vi "自动售货机.vi"() -> ()   [LabVIEW 2018]
panel:
  in  "数值 2":dbl
  in  "数值":dbl
  in  "选项卡控件":enum32{"前面板", "后台"}(tab)
  in  "果粒橙":bool
  in  "营养快线":bool
  in  "矿泉水":bool
  in  "花生奶":bool
  in  "绿茶":bool
  in  "雪梨":bool
  in  "红牛":bool
  in  "八宝粥":bool
  in  "王老吉":bool
  in  "可乐":bool
  in  "雪碧":bool
  in  "百事":bool
  in  "退币":bool
  in  "5角":bool
  in  "1元":bool
  in  "5元":bool
  in  "10元":bool
  in  "投币显示":string
  in  "字符串":string
  out "果粒橙":dbl
  out "营养快线":dbl
  out "矿泉水":dbl
  out "花生奶":dbl
  out "绿茶":dbl
  out "雪梨":dbl
  out "红牛":dbl
  out "八宝粥":dbl
  out "王老吉":dbl
  out "可乐":dbl
  out "雪碧":dbl
  out "百事":dbl
  in  "销售金额":string
  in  "关闭售货机":bool
  in  "销售记录":string
  in  "果粒橙单价":dbl
  in  "营养快线数量":dbl
  in  "矿泉水数量":dbl
  in  "花生奶数量":dbl
  in  "绿茶数量":dbl
  in  "雪梨数量":dbl
  in  "红牛数量":dbl
  in  "八宝粥数量":dbl
  in  "王老吉数量":dbl
  in  "可乐数量":dbl
  in  "雪碧数量":dbl
  in  "百事数量":dbl
  in  "果粒橙数量":dbl
  in  "营养快线单价":dbl
  in  "矿泉水单价":dbl
  in  "花生奶单价":dbl
  in  "绿茶单价":dbl
  in  "雪梨单价":dbl
  in  "红牛单价":dbl
  in  "八宝粥单价":dbl
  in  "王老吉单价":dbl
  in  "可乐单价":dbl
  in  "雪碧单价":dbl
  in  "上货":bool
  in  "百事单价":dbl
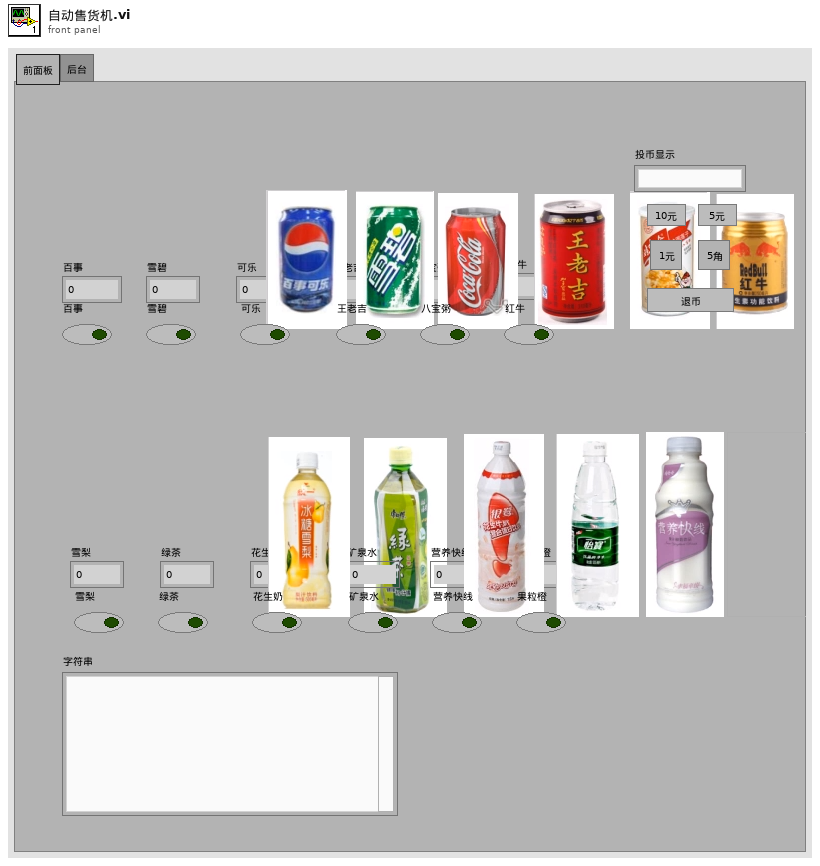
[diagram p1: front panel]
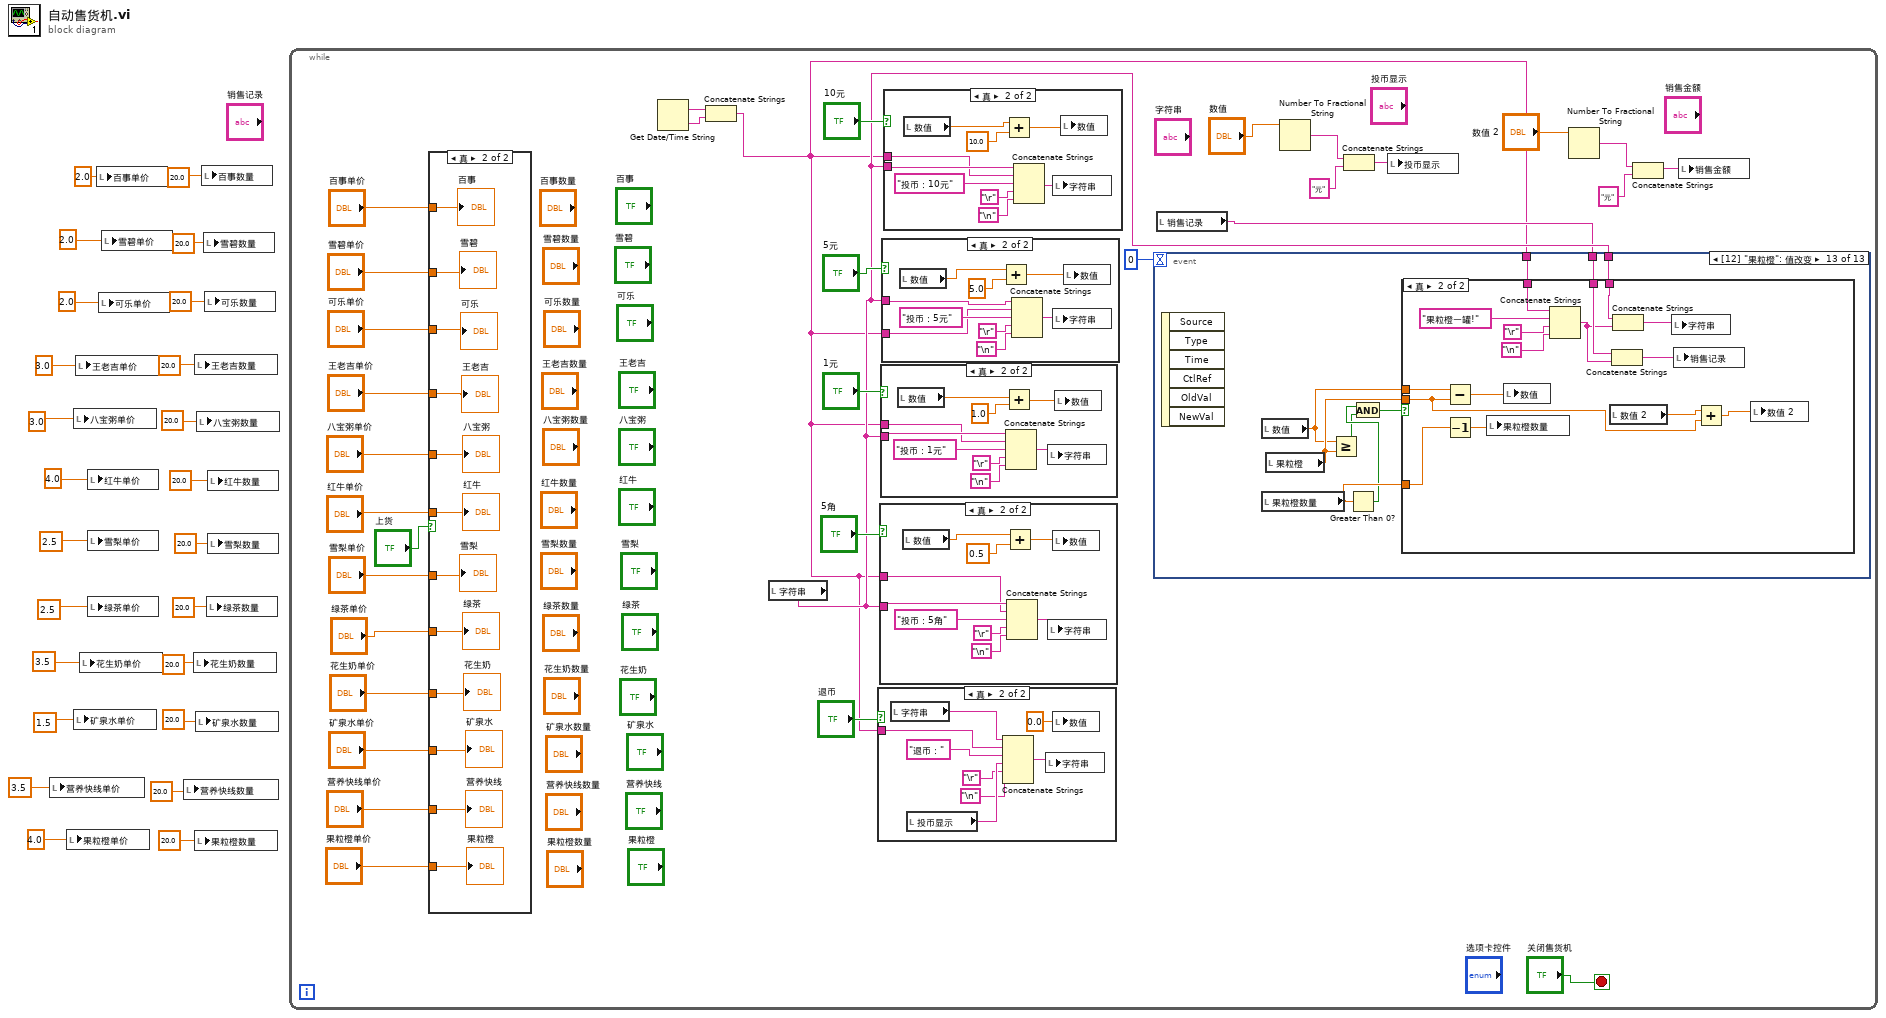
[diagram p0: block diagram]
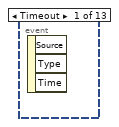
[diagram p2: hidden frame]
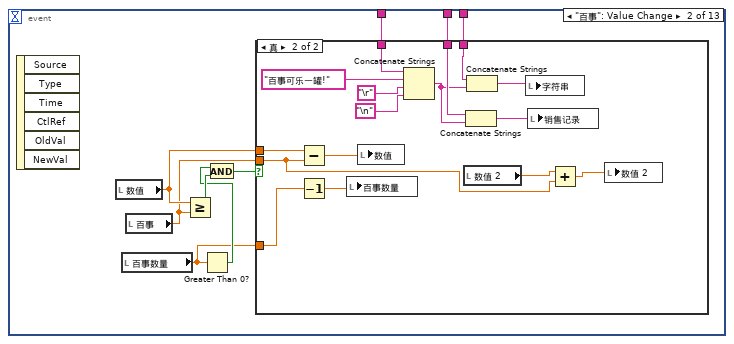
[diagram p3: hidden frame]
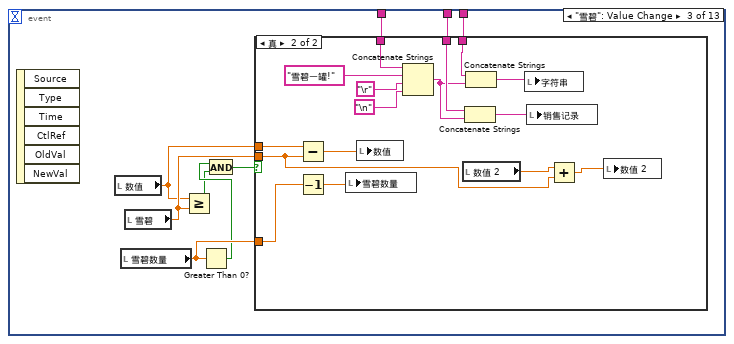
[diagram p5: hidden frame]
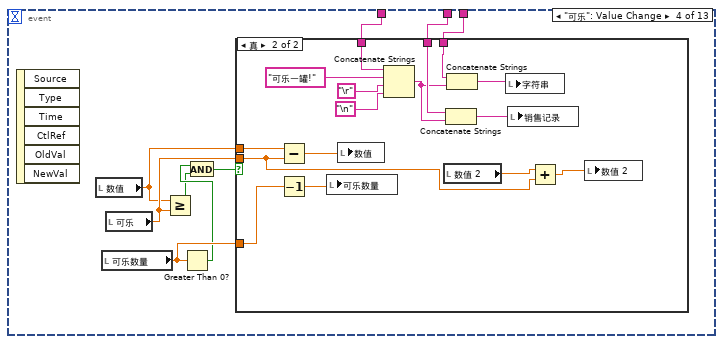
[diagram p7: hidden frame]
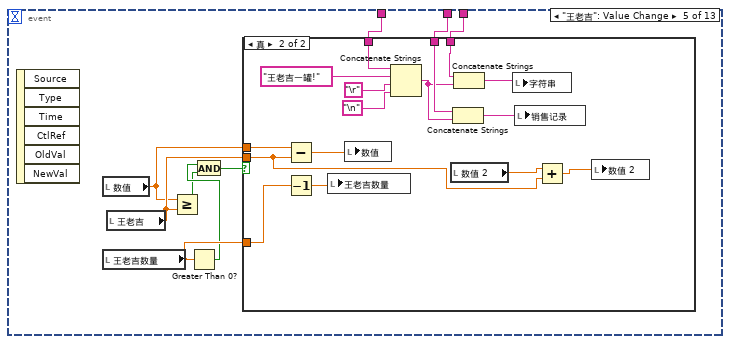
[diagram p9: hidden frame]
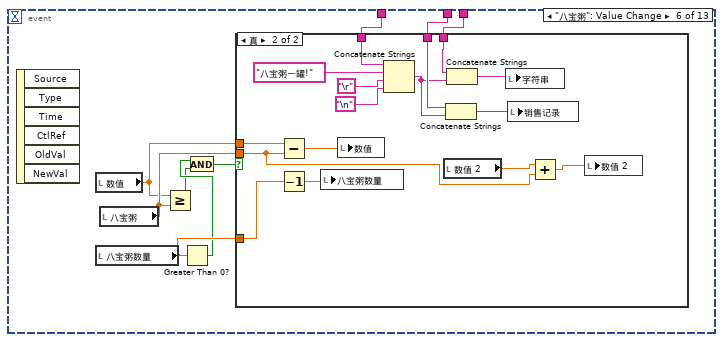
[diagram p11: hidden frame]
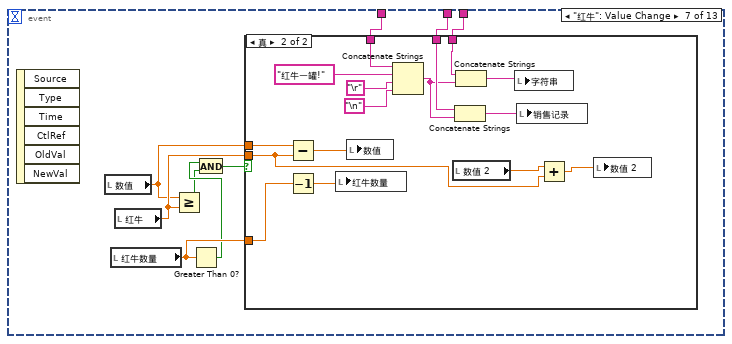
[diagram p13: hidden frame]
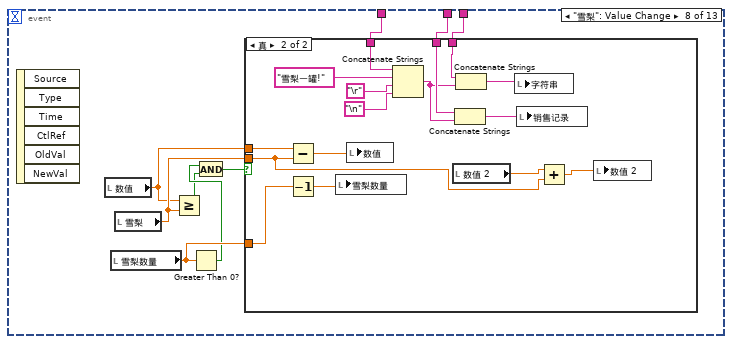
[diagram p15: hidden frame]
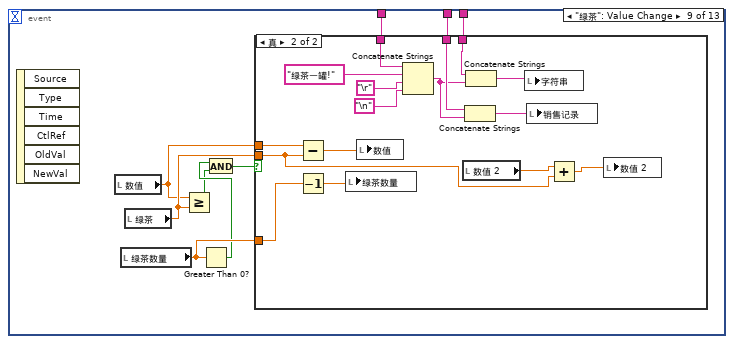
[diagram p17: hidden frame]
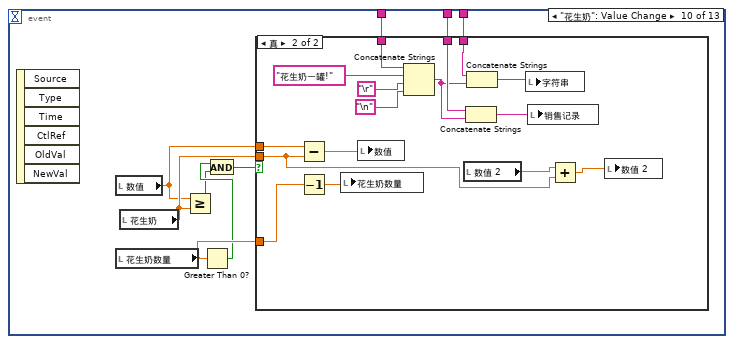
[diagram p19: hidden frame]
diagram:
  n1 = local write "营养快线单价"(3.5 ("百事单价")) -> ()
  n2 = local write "果粒橙单价"(4.0 ("百事单价")) -> ()
  n3 = local write "八宝粥单价"(3.0 ("百事单价")) -> ()
  n4 = local write "矿泉水单价"(1.5 ("百事单价")) -> ()
  n5 = local write "王老吉单价"(3.0 ("百事单价")) -> ()
  n6 = local write "花生奶单价"(3.5 ("百事单价")) -> ()
  n7 = local write "红牛单价"(4.0 ("百事单价")) -> ()
  n8 = local write "雪梨单价"(2.5 ("百事单价")) -> ()
  n9 = local write "绿茶单价"(2.5 ("百事单价")) -> ()
  n10 = local write "百事单价"(2.0 ("百事单价")) -> ()
  n11 = local write "可乐单价"(2.0 ("百事单价")) -> ()
  n12 = local write "雪碧单价"(2.0 ("百事单价")) -> ()
  n13 = local write "营养快线数量"(20.0 ("百事单价")) -> ()
  n14 = local write "花生奶数量"(20.0 ("百事单价")) -> ()
  n15 = local write "王老吉数量"(20.0 ("百事单价")) -> ()
  n16 = local write "果粒橙数量"(20.0 ("百事单价")) -> ()
  n17 = local write "矿泉水数量"(20.0 ("百事单价")) -> ()
  n18 = local write "八宝粥数量"(20.0 ("百事单价")) -> ()
  n19 = local write "百事数量"(20.0 ("百事单价")) -> ()
  n20 = local write "雪碧数量"(20.0 ("百事单价")) -> ()
  n21 = local write "可乐数量"(20.0 ("百事单价")) -> ()
  n22 = local write "绿茶数量"(20.0 ("百事单价")) -> ()
  n23 = local write "红牛数量"(20.0 ("百事单价")) -> ()
  n24 = local write "雪梨数量"(20.0 ("百事单价")) -> ()
  n25 = while {
    stop <- "关闭售货机" stop-if-true
    n26 = case shown="真" "上货" {
      tunnel: "百事单价" -> [_ w413]
      tunnel: "雪碧单价" -> [_ w412]
      tunnel: "可乐单价" -> [_ w411]
      tunnel: "王老吉单价" -> [_ w410]
      tunnel: "八宝粥单价" -> [_ w409]
      tunnel: "红牛单价" -> [_ w408]
      tunnel: "雪梨单价" -> [_ w407]
      tunnel: "绿茶单价" -> [_ w406]
      tunnel: "花生奶单价" -> [_ w405]
      tunnel: "矿泉水单价" -> [_ w404]
      tunnel: "营养快线单价" -> [_ w403]
      tunnel: "果粒橙单价" -> [_ w402]
      frame False {
      }
      frame True {
        "百事" <- w413
        "雪碧" <- w412
        "可乐" <- w411
        "王老吉" <- w410
        "八宝粥" <- w409
        "红牛" <- w408
        "雪梨" <- w407
        "绿茶" <- w406
        "花生奶" <- w405
        "矿泉水" <- w404
        "营养快线" <- w403
        "果粒橙" <- w402
      }
    }
    n27 = Get Date/Time String() -> (date string=w29:string, time string=w28:string)  [unwired: 3 in]
    n28 = Concatenate Strings(w29, w28) -> (w27:string)
    n29 = local read "字符串"() -> (w34:string)
    n30 = case shown="真" "退币" {
      tunnel: w27 -> [_ w358]
      frame False {
      }
      frame True {
        n31 = local read "字符串"() -> (w359:string)
        n32 = local read "投币显示"() -> (w362:string)
        n33 = Concatenate Strings(w359, w358, "退币：" ("字符串"), w362, "\r", "\n") -> (w364:string)
        n34 = local write "字符串"(w364) -> ()
        n35 = local write "数值"(0.0 ("数值")) -> ()
      }
    }
    n36 = case shown="真" "5角" {
      tunnel: w34 -> [_ w367]
      tunnel: w27 -> [_ w366]
      frame False {
      }
      frame True {
        n37 = local read "数值"() -> (w372:dbl)
        n38 = Add(x=w372, y=0.5) -> (x+y=w373:dbl)
        n39 = Concatenate Strings(w367, w366, "投币：5角" ("字符串"), "\r", "\n") -> (w371:string)
        n40 = local write "字符串"(w371) -> ()
        n41 = local write "数值"(w373) -> ()
      }
    }
    n42 = case shown="真" "1元" {
      tunnel: w34 -> [_ w376]
      tunnel: w27 -> [_ w375]
      frame False {
      }
      frame True {
        n43 = local read "数值"() -> (w381:dbl)
        n44 = Add(x=w381, y=1.0) -> (x+y=w382:dbl)
        n45 = Concatenate Strings(w376, w375, "投币：1元" ("字符串"), "\r", "\n") -> (w377:string)
        n46 = local write "字符串"(w377) -> ()
        n47 = local write "数值"(w382) -> ()
      }
    }
    n48 = case shown="真" "5元" {
      tunnel: w34 -> [_ w385]
      tunnel: w27 -> [_ w384]
      frame False {
      }
      frame True {
        n49 = local read "数值"() -> (w390:dbl)
        n50 = Add(x=w390, y=5.0) -> (x+y=w391:dbl)
        n51 = Concatenate Strings(w385, w384, "投币：5元" ("字符串"), "\r", "\n") -> (w386:string)
        n52 = local write "字符串"(w386) -> ()
        n53 = local write "数值"(w391) -> ()
      }
    }
    n54 = case shown="真" "10元" {
      tunnel: w34 -> [_ w394]
      tunnel: w27 -> [_ w393]
      frame False {
      }
      frame True {
        n55 = local read "数值"() -> (w400:dbl)
        n56 = Add(x=w400, y=10.0) -> (x+y=w401:dbl)
        n57 = Concatenate Strings(w394, w393, "投币：10元" ("字符串"), "\r", "\n") -> (w395:string)
        n58 = local write "字符串"(w395) -> ()
        n59 = local write "数值"(w401) -> ()
      }
    }
    n60 = local read "销售记录"() -> (w33:string)
    n61 = event shown="[12] \"果粒橙\": 值改变" {
      selector: _ -> [_ _ _ _ _ _ _ _ _ _ _ _ _]
      dyn-events: _ -> [_ _ _ _ _ _ _ _ _ _ _ _ _]
      timeout: 0 -> [_ _ _ _ _ _ _ _ _ _ _ _ _]
      tunnel: w34 -> [_ w66 w85 w110 w134 w160 w183 w209 w235 w258 w285 w310 w335]
      tunnel: w33 -> [_ w65 w84 w109 w135 w159 w184 w210 w234 w259 w284 w309 w334]
      tunnel: w27 -> [_ w58 w83 w108 w133 w158 w185 w208 w233 w260 w283 w308 w333]
      event Timeout {
        n62 = event-data() -> ()  [unwired: 1 in, 3 out]
      }
      event "百事": Value Change {
        n63 = event-data() -> ()  [unwired: 1 in, 6 out]
        n64 = local read "数值"() -> (w64:dbl)
        n65 = local read "百事数量"() -> (w59:dbl)
        n66 = local read "百事"() -> (w63:dbl)
        n67 = Greater Or Equal?(x=w64, y=w63) -> (x >= y?=w62:bool)
        n68 = Greater Than 0?(x=w59) -> (x > 0?=w60:bool)
        n69 = And(x=w60, y=w62) -> (x .and. y?=w61:bool)
        n70 = case shown="真" w61 {
          tunnel: w66 -> [_ w78]
          tunnel: w65 -> [_ w77]
          tunnel: w64 -> [_ w74]
          tunnel: w63 -> [_ w69]
          tunnel: w59 -> [_ w72]
          tunnel: w58 -> [_ w68]
          frame False {
          }
          frame True {
            n71 = Subtract(x=w74, y=w69) -> (x-y=w75:dbl)
            n72 = Decrement(x=w72) -> (x-1=w73:dbl)
            n73 = local write "百事数量"(w73) -> ()
            n74 = local write "数值"(w75) -> ()
            n75 = Concatenate Strings(w68, "百事可乐一罐!" ("字符串"), "\r", "\n") -> (w76:string)
            n76 = local read "数值 2"() -> (w71:dbl)
            n77 = Concatenate Strings(w77, w76) -> (w67:string)
            n78 = Concatenate Strings(w78, w76) -> (w79:string)
            n79 = local write "字符串"(w79) -> ()
            n80 = local write "销售记录"(w67) -> ()
            n81 = Add(x=w71, y=w69) -> (x+y=w70:dbl)
            n82 = local write "数值 2"(w70) -> ()
          }
        }
      }
      event "雪碧": Value Change {
        n83 = event-data() -> ()  [unwired: 1 in, 6 out]
        n84 = local read "数值"() -> (w86:dbl)
        n85 = local read "雪碧数量"() -> (w91:dbl)
        n86 = local read "雪碧"() -> (w87:dbl)
        n87 = Greater Or Equal?(x=w86, y=w87) -> (x >= y?=w88:bool)
        n88 = Greater Than 0?(x=w91) -> (x > 0?=w90:bool)
        n89 = And(x=w90, y=w88) -> (x .and. y?=w89:bool)
        n90 = case shown="真" w89 {
          tunnel: w85 -> [_ w103]
          tunnel: w84 -> [_ w102]
          tunnel: w86 -> [_ w99]
          tunnel: w87 -> [_ w94]
          tunnel: w91 -> [_ w97]
          tunnel: w83 -> [_ w93]
          frame False {
          }
          frame True {
            n91 = Subtract(x=w99, y=w94) -> (x-y=w100:dbl)
            n92 = Decrement(x=w97) -> (x-1=w98:dbl)
            n93 = local write "雪碧数量"(w98) -> ()
            n94 = local write "数值"(w100) -> ()
            n95 = Concatenate Strings(w93, "雪碧一罐!" ("字符串"), "\r", "\n") -> (w101:string)
            n96 = local read "数值 2"() -> (w96:dbl)
            n97 = Concatenate Strings(w102, w101) -> (w92:string)
            n98 = Concatenate Strings(w103, w101) -> (w104:string)
            n99 = local write "字符串"(w104) -> ()
            n100 = local write "销售记录"(w92) -> ()
            n101 = Add(x=w96, y=w94) -> (x+y=w95:dbl)
            n102 = local write "数值 2"(w95) -> ()
          }
        }
      }
      event "可乐": Value Change {
        n103 = event-data() -> ()  [unwired: 1 in, 6 out]
        n104 = local read "数值"() -> (w111:dbl)
        n105 = local read "可乐数量"() -> (w116:dbl)
        n106 = local read "可乐"() -> (w112:dbl)
        n107 = Greater Or Equal?(x=w111, y=w112) -> (x >= y?=w113:bool)
        n108 = Greater Than 0?(x=w116) -> (x > 0?=w115:bool)
        n109 = And(x=w115, y=w113) -> (x .and. y?=w114:bool)
        n110 = case shown="真" w114 {
          tunnel: w110 -> [_ w128]
          tunnel: w109 -> [_ w127]
          tunnel: w111 -> [_ w124]
          tunnel: w112 -> [_ w119]
          tunnel: w116 -> [_ w122]
          tunnel: w108 -> [_ w118]
          frame False {
          }
          frame True {
            n111 = Subtract(x=w124, y=w119) -> (x-y=w125:dbl)
            n112 = Decrement(x=w122) -> (x-1=w123:dbl)
            n113 = local write "可乐数量"(w123) -> ()
            n114 = local write "数值"(w125) -> ()
            n115 = Concatenate Strings(w118, "可乐一罐!" ("字符串"), "\r", "\n") -> (w126:string)
            n116 = local read "数值 2"() -> (w121:dbl)
            n117 = Concatenate Strings(w127, w126) -> (w117:string)
            n118 = Concatenate Strings(w128, w126) -> (w129:string)
            n119 = local write "字符串"(w129) -> ()
            n120 = local write "销售记录"(w117) -> ()
            n121 = Add(x=w121, y=w119) -> (x+y=w120:dbl)
            n122 = local write "数值 2"(w120) -> ()
          }
        }
      }
      event "王老吉": Value Change {
        n123 = event-data() -> ()  [unwired: 1 in, 6 out]
        n124 = local read "数值"() -> (w136:dbl)
        n125 = local read "王老吉数量"() -> (w141:dbl)
        n126 = local read "王老吉"() -> (w137:dbl)
        n127 = Greater Or Equal?(x=w136, y=w137) -> (x >= y?=w138:bool)
        n128 = Greater Than 0?(x=w141) -> (x > 0?=w140:bool)
        n129 = And(x=w140, y=w138) -> (x .and. y?=w139:bool)
        n130 = case shown="真" w139 {
          tunnel: w134 -> [_ w153]
          tunnel: w135 -> [_ w152]
          tunnel: w136 -> [_ w149]
          tunnel: w137 -> [_ w144]
          tunnel: w141 -> [_ w147]
          tunnel: w133 -> [_ w143]
          frame False {
          }
          frame True {
            n131 = Subtract(x=w149, y=w144) -> (x-y=w150:dbl)
            n132 = Decrement(x=w147) -> (x-1=w148:dbl)
            n133 = local write "王老吉数量"(w148) -> ()
            n134 = local write "数值"(w150) -> ()
            n135 = Concatenate Strings(w143, "王老吉一罐!" ("字符串"), "\r", "\n") -> (w151:string)
            n136 = local read "数值 2"() -> (w146:dbl)
            n137 = Concatenate Strings(w152, w151) -> (w142:string)
            n138 = Concatenate Strings(w153, w151) -> (w154:string)
            n139 = local write "字符串"(w154) -> ()
            n140 = local write "销售记录"(w142) -> ()
            n141 = Add(x=w146, y=w144) -> (x+y=w145:dbl)
            n142 = local write "数值 2"(w145) -> ()
          }
        }
      }
      event "八宝粥": Value Change {
        n143 = event-data() -> ()  [unwired: 1 in, 6 out]
        n144 = local read "数值"() -> (w161:dbl)
        n145 = local read "八宝粥数量"() -> (w166:dbl)
        n146 = local read "八宝粥"() -> (w162:dbl)
        n147 = Greater Or Equal?(x=w161, y=w162) -> (x >= y?=w163:bool)
        n148 = Greater Than 0?(x=w166) -> (x > 0?=w165:bool)
        n149 = And(x=w165, y=w163) -> (x .and. y?=w164:bool)
        n150 = case shown="真" w164 {
          tunnel: w160 -> [_ w178]
          tunnel: w159 -> [_ w177]
          tunnel: w161 -> [_ w174]
          tunnel: w162 -> [_ w169]
          tunnel: w166 -> [_ w172]
          tunnel: w158 -> [_ w168]
          frame False {
          }
          frame True {
            n151 = Subtract(x=w174, y=w169) -> (x-y=w175:dbl)
            n152 = Decrement(x=w172) -> (x-1=w173:dbl)
            n153 = local write "八宝粥数量"(w173) -> ()
            n154 = local write "数值"(w175) -> ()
            n155 = Concatenate Strings(w168, "八宝粥一罐!" ("字符串"), "\r", "\n") -> (w176:string)
            n156 = local read "数值 2"() -> (w171:dbl)
            n157 = Concatenate Strings(w177, w176) -> (w167:string)
            n158 = Concatenate Strings(w178, w176) -> (w179:string)
            n159 = local write "字符串"(w179) -> ()
            n160 = local write "销售记录"(w167) -> ()
            n161 = Add(x=w171, y=w169) -> (x+y=w170:dbl)
            n162 = local write "数值 2"(w170) -> ()
          }
        }
      }
      event "红牛": Value Change {
        n163 = event-data() -> ()  [unwired: 1 in, 6 out]
        n164 = local read "数值"() -> (w186:dbl)
        n165 = local read "红牛数量"() -> (w191:dbl)
        n166 = local read "红牛"() -> (w187:dbl)
        n167 = Greater Or Equal?(x=w186, y=w187) -> (x >= y?=w188:bool)
        n168 = Greater Than 0?(x=w191) -> (x > 0?=w190:bool)
        n169 = And(x=w190, y=w188) -> (x .and. y?=w189:bool)
        n170 = case shown="真" w189 {
          tunnel: w183 -> [_ w203]
          tunnel: w184 -> [_ w202]
          tunnel: w186 -> [_ w199]
          tunnel: w187 -> [_ w194]
          tunnel: w191 -> [_ w197]
          tunnel: w185 -> [_ w193]
          frame False {
          }
          frame True {
            n171 = Subtract(x=w199, y=w194) -> (x-y=w200:dbl)
            n172 = Decrement(x=w197) -> (x-1=w198:dbl)
            n173 = local write "红牛数量"(w198) -> ()
            n174 = local write "数值"(w200) -> ()
            n175 = Concatenate Strings(w193, "红牛一罐!" ("字符串"), "\r", "\n") -> (w201:string)
            n176 = local read "数值 2"() -> (w196:dbl)
            n177 = Concatenate Strings(w202, w201) -> (w192:string)
            n178 = Concatenate Strings(w203, w201) -> (w204:string)
            n179 = local write "字符串"(w204) -> ()
            n180 = local write "销售记录"(w192) -> ()
            n181 = Add(x=w196, y=w194) -> (x+y=w195:dbl)
            n182 = local write "数值 2"(w195) -> ()
          }
        }
      }
      event "雪梨": Value Change {
        n183 = event-data() -> ()  [unwired: 1 in, 6 out]
        n184 = local read "数值"() -> (w211:dbl)
        n185 = local read "雪梨数量"() -> (w216:dbl)
        n186 = local read "雪梨"() -> (w212:dbl)
        n187 = Greater Or Equal?(x=w211, y=w212) -> (x >= y?=w213:bool)
        n188 = Greater Than 0?(x=w216) -> (x > 0?=w215:bool)
        n189 = And(x=w215, y=w213) -> (x .and. y?=w214:bool)
        n190 = case shown="真" w214 {
          tunnel: w209 -> [_ w228]
          tunnel: w210 -> [_ w227]
          tunnel: w211 -> [_ w224]
          tunnel: w212 -> [_ w219]
          tunnel: w216 -> [_ w222]
          tunnel: w208 -> [_ w218]
          frame False {
          }
          frame True {
            n191 = Subtract(x=w224, y=w219) -> (x-y=w225:dbl)
            n192 = Decrement(x=w222) -> (x-1=w223:dbl)
            n193 = local write "雪梨数量"(w223) -> ()
            n194 = local write "数值"(w225) -> ()
            n195 = Concatenate Strings(w218, "雪梨一罐!" ("字符串"), "\r", "\n") -> (w226:string)
            n196 = local read "数值 2"() -> (w221:dbl)
            n197 = Concatenate Strings(w227, w226) -> (w217:string)
            n198 = Concatenate Strings(w228, w226) -> (w229:string)
            n199 = local write "字符串"(w229) -> ()
            n200 = local write "销售记录"(w217) -> ()
            n201 = Add(x=w221, y=w219) -> (x+y=w220:dbl)
            n202 = local write "数值 2"(w220) -> ()
          }
        }
      }
      event "绿茶": Value Change {
        n203 = event-data() -> ()  [unwired: 1 in, 6 out]
        n204 = local read "数值"() -> (w236:dbl)
        n205 = local read "绿茶数量"() -> (w241:dbl)
        n206 = local read "绿茶"() -> (w237:dbl)
        n207 = Greater Or Equal?(x=w236, y=w237) -> (x >= y?=w238:bool)
        n208 = Greater Than 0?(x=w241) -> (x > 0?=w240:bool)
        n209 = And(x=w240, y=w238) -> (x .and. y?=w239:bool)
        n210 = case shown="真" w239 {
          tunnel: w235 -> [_ w253]
          tunnel: w234 -> [_ w252]
          tunnel: w236 -> [_ w249]
          tunnel: w237 -> [_ w244]
          tunnel: w241 -> [_ w247]
          tunnel: w233 -> [_ w243]
          frame False {
          }
          frame True {
            n211 = Subtract(x=w249, y=w244) -> (x-y=w250:dbl)
            n212 = Decrement(x=w247) -> (x-1=w248:dbl)
            n213 = local write "绿茶数量"(w248) -> ()
            n214 = local write "数值"(w250) -> ()
            n215 = Concatenate Strings(w243, "绿茶一罐!" ("字符串"), "\r", "\n") -> (w251:string)
            n216 = local read "数值 2"() -> (w246:dbl)
            n217 = Concatenate Strings(w252, w251) -> (w242:string)
            n218 = Concatenate Strings(w253, w251) -> (w254:string)
            n219 = local write "字符串"(w254) -> ()
            n220 = local write "销售记录"(w242) -> ()
            n221 = Add(x=w246, y=w244) -> (x+y=w245:dbl)
            n222 = local write "数值 2"(w245) -> ()
          }
        }
      }
      event "花生奶": Value Change {
        n223 = event-data() -> ()  [unwired: 1 in, 6 out]
        n224 = local read "数值"() -> (w261:dbl)
        n225 = local read "花生奶数量"() -> (w266:dbl)
        n226 = local read "花生奶"() -> (w262:dbl)
        n227 = Greater Or Equal?(x=w261, y=w262) -> (x >= y?=w263:bool)
        n228 = Greater Than 0?(x=w266) -> (x > 0?=w265:bool)
        n229 = And(x=w265, y=w263) -> (x .and. y?=w264:bool)
        n230 = case shown="真" w264 {
          tunnel: w258 -> [_ w278]
          tunnel: w259 -> [_ w277]
          tunnel: w261 -> [_ w274]
          tunnel: w262 -> [_ w269]
          tunnel: w266 -> [_ w272]
          tunnel: w260 -> [_ w268]
          frame False {
          }
          frame True {
            n231 = Subtract(x=w274, y=w269) -> (x-y=w275:dbl)
            n232 = Decrement(x=w272) -> (x-1=w273:dbl)
            n233 = local write "花生奶数量"(w273) -> ()
            n234 = local write "数值"(w275) -> ()
            n235 = Concatenate Strings(w268, "花生奶一罐!" ("字符串"), "\r", "\n") -> (w276:string)
            n236 = local read "数值 2"() -> (w271:dbl)
            n237 = Concatenate Strings(w277, w276) -> (w267:string)
            n238 = Concatenate Strings(w278, w276) -> (w279:string)
            n239 = local write "字符串"(w279) -> ()
            n240 = local write "销售记录"(w267) -> ()
            n241 = Add(x=w271, y=w269) -> (x+y=w270:dbl)
            n242 = local write "数值 2"(w270) -> ()
          }
        }
      }
      event "矿泉水": Value Change {
        n243 = event-data() -> ()  [unwired: 1 in, 6 out]
        n244 = local read "数值"() -> (w286:dbl)
        n245 = local read "矿泉水数量"() -> (w291:dbl)
        n246 = local read "矿泉水"() -> (w287:dbl)
        n247 = Greater Or Equal?(x=w286, y=w287) -> (x >= y?=w288:bool)
        n248 = Greater Than 0?(x=w291) -> (x > 0?=w290:bool)
        n249 = And(x=w290, y=w288) -> (x .and. y?=w289:bool)
        n250 = case shown="真" w289 {
          tunnel: w285 -> [_ w303]
          tunnel: w284 -> [_ w302]
          tunnel: w286 -> [_ w299]
          tunnel: w287 -> [_ w294]
          tunnel: w291 -> [_ w297]
          tunnel: w283 -> [_ w293]
          frame False {
          }
          frame True {
            n251 = Subtract(x=w299, y=w294) -> (x-y=w300:dbl)
            n252 = Decrement(x=w297) -> (x-1=w298:dbl)
            n253 = local write "矿泉水数量"(w298) -> ()
            n254 = local write "数值"(w300) -> ()
            n255 = Concatenate Strings(w293, "矿泉水一瓶!" ("字符串"), "\r", "\n") -> (w301:string)
            n256 = local read "数值 2"() -> (w296:dbl)
            n257 = Concatenate Strings(w302, w301) -> (w292:string)
            n258 = Concatenate Strings(w303, w301) -> (w304:string)
            n259 = local write "字符串"(w304) -> ()
            n260 = local write "销售记录"(w292) -> ()
            n261 = Add(x=w296, y=w294) -> (x+y=w295:dbl)
            n262 = local write "数值 2"(w295) -> ()
          }
        }
      }
      event "营养快线": Value Change {
        n263 = event-data() -> ()  [unwired: 1 in, 6 out]
        n264 = local read "营养快线数量"() -> (w316:dbl)
        n265 = local read "营养快线"() -> (w312:dbl)
        n266 = local read "数值"() -> (w311:dbl)
        n267 = Greater Or Equal?(x=w311, y=w312) -> (x >= y?=w313:bool)
        n268 = Greater Than 0?(x=w316) -> (x > 0?=w315:bool)
        n269 = And(x=w315, y=w313) -> (x .and. y?=w314:bool)
        n270 = case shown="真" w314 {
          tunnel: w310 -> [_ w328]
          tunnel: w309 -> [_ w327]
          tunnel: w311 -> [_ w324]
          tunnel: w312 -> [_ w319]
          tunnel: w316 -> [_ w322]
          tunnel: w308 -> [_ w318]
          frame False {
          }
          frame True {
            n271 = Subtract(x=w324, y=w319) -> (x-y=w325:dbl)
            n272 = Decrement(x=w322) -> (x-1=w323:dbl)
            n273 = local write "营养快线数量"(w323) -> ()
            n274 = local write "数值"(w325) -> ()
            n275 = Concatenate Strings(w318, "营养快线一罐!" ("字符串"), "\r", "\n") -> (w326:string)
            n276 = local read "数值 2"() -> (w321:dbl)
            n277 = Concatenate Strings(w327, w326) -> (w317:string)
            n278 = Concatenate Strings(w328, w326) -> (w329:string)
            n279 = local write "字符串"(w329) -> ()
            n280 = local write "销售记录"(w317) -> ()
            n281 = Add(x=w321, y=w319) -> (x+y=w320:dbl)
            n282 = local write "数值 2"(w320) -> ()
          }
        }
      }
      event "果粒橙": Value Change {
        n283 = event-data() -> ()  [unwired: 1 in, 6 out]
        n284 = local read "数值"() -> (w336:dbl)
        n285 = local read "果粒橙数量"() -> (w341:dbl)
        n286 = local read "果粒橙"() -> (w337:dbl)
        n287 = Greater Or Equal?(x=w336, y=w337) -> (x >= y?=w338:bool)
        n288 = Greater Than 0?(x=w341) -> (x > 0?=w340:bool)
        n289 = And(x=w340, y=w338) -> (x .and. y?=w339:bool)
        n290 = case shown="真" w339 {
          tunnel: w335 -> [_ w353]
          tunnel: w334 -> [_ w352]
          tunnel: w336 -> [_ w349]
          tunnel: w337 -> [_ w344]
          tunnel: w341 -> [_ w347]
          tunnel: w333 -> [_ w343]
          frame False {
          }
          frame True {
            n291 = Subtract(x=w349, y=w344) -> (x-y=w350:dbl)
            n292 = Decrement(x=w347) -> (x-1=w348:dbl)
            n293 = local write "果粒橙数量"(w348) -> ()
            n294 = local write "数值"(w350) -> ()
            n295 = Concatenate Strings(w343, "果粒橙一罐!" ("字符串"), "\r", "\n") -> (w351:string)
            n296 = local read "数值 2"() -> (w346:dbl)
            n297 = Concatenate Strings(w352, w351) -> (w342:string)
            n298 = Concatenate Strings(w353, w351) -> (w354:string)
            n299 = local write "字符串"(w354) -> ()
            n300 = local write "销售记录"(w342) -> ()
            n301 = Add(x=w346, y=w344) -> (x+y=w345:dbl)
            n302 = local write "数值 2"(w345) -> ()
          }
        }
      }
    }
    n303 = Number To Fractional String(number="数值") -> (F-format string=w42:string)  [unwired: 3 in]
    n304 = Concatenate Strings(w42, "元" ("字符串")) -> (w26:string)
    n305 = local write "投币显示"(w26) -> ()
    n306 = Number To Fractional String(number="数值 2") -> (F-format string=w31:string)  [unwired: 3 in]
    n307 = Concatenate Strings(w31, "元" ("字符串")) -> (w25:string)
    n308 = local write "销售金额"(w25) -> ()
  }
